vi "sub.vi"   [LabVIEW 2025, in "Demo1.lvlib"]
uses:
  Demo1.lvlib
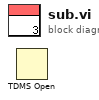
[diagram p0: block diagram]
diagram:
  n1 = TDMS Open() -> ()  [unwired: 7 in, 2 out]
